vi "j.vi"() -> ()   [LabVIEW 2020]
panel:
  out "Output_Array":u32[](array[numeric])
  in  "Dot_Color 2":u32(colorbox)
  in  "Dot_Color":u32(colorbox)
  in  "Trail_Length":dbl
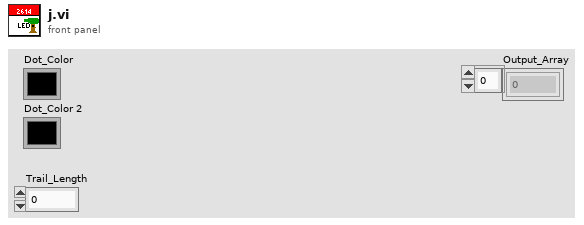
[diagram p1: front panel]
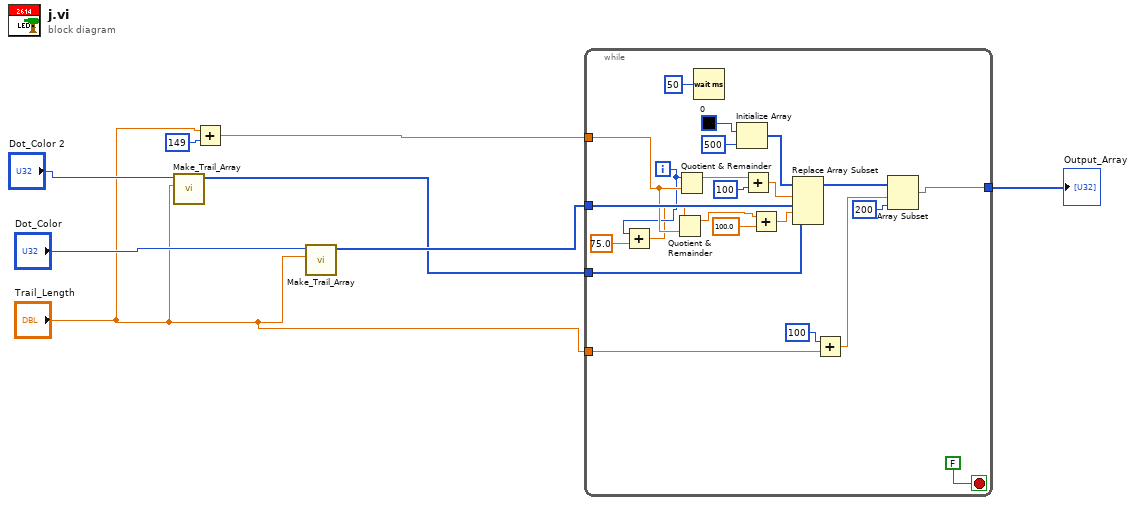
[diagram p0: block diagram]
diagram:
  n1 = call "Make_Trail_Array.vi"("Trail_Length"="Trail_Length", "Dot_Color"="Dot_Color 2") -> ("Trail_Array"=w2:u32[])  [unwired: 9 in]
  n2 = Add(x="Trail_Length", y=149 ("x")) -> (x+y=w5:dbl)
  n3 = call "Make_Trail_Array.vi"("Trail_Length"="Trail_Length", "Dot_Color"="Dot_Color") -> ("Trail_Array"=w7:u32[])  [unwired: 9 in]
  n4 = while {
    tunnel: w7 -> [w19]
    tunnel: "Trail_Length" -> [w21]
    tunnel: w5 -> [w13]
    tunnel: w2 -> [w10]
    tunnel: [w9] -> w1
    i -> [w12]
    stop <- FALSE stop-if-true
    n5 = Add(x=w12, y=75.0) -> (x+y=w11:dbl)
    n6 = Quotient & Remainder(x=w11, y=w13) -> (x-y*floor(x/y)=w14:dbl)  [unwired: 1 out]
    n7 = Quotient & Remainder(x=w12, y=w13) -> (x-y*floor(x/y)=w18:dbl)  [unwired: 1 out]
    n8 = Wait (ms)(milliseconds to wait=u32 50) -> ()  [unwired: 1 out]
    n9 = Initialize Array(u32 0, 500 ("dimension size")) -> (w27:u32[])
    n10 = Add(x=w18, y=100) -> (x+y=w23:dbl)
    n11 = Add(x=w14, y=100.0) -> (x+y=w16:dbl)
    n12 = Replace Array Subset(array=w27, new element #1=w19, index #1=w23, new element #2=w10, index #2=w16) -> (w26:u32[])
    n13 = Add(x=100 ("index"), y=w21) -> (x+y=w20:dbl)
    n14 = Array Subset(array=w26, index=w20, length=200) -> (w9:u32[])
  }
  "Output_Array" <- w1
